vi "电源管理UI.vi"() -> ()   [LabVIEW 2016, in "PLC.lvlib"]
uses:
  PLC.lvlib
  <vilib>/Utility/miscctls.llb/LVPointTypeDef.ctl
panel:
  in  "自动运行启动参数":T1
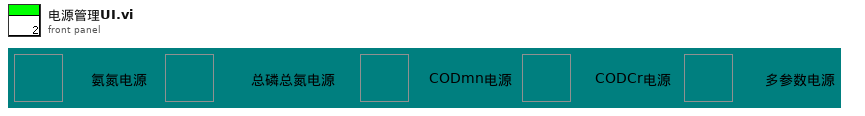
[diagram p1: front panel]
types:
  T1 = cluster{"氨氮":bool, "总磷总氮":bool, "CODmn":bool, "CODCr":bool, "多参数":bool}
  T2 = typedef "LVPointTypeDef.ctl" = cluster{"Horizontal":i16, "Vertical":i16}
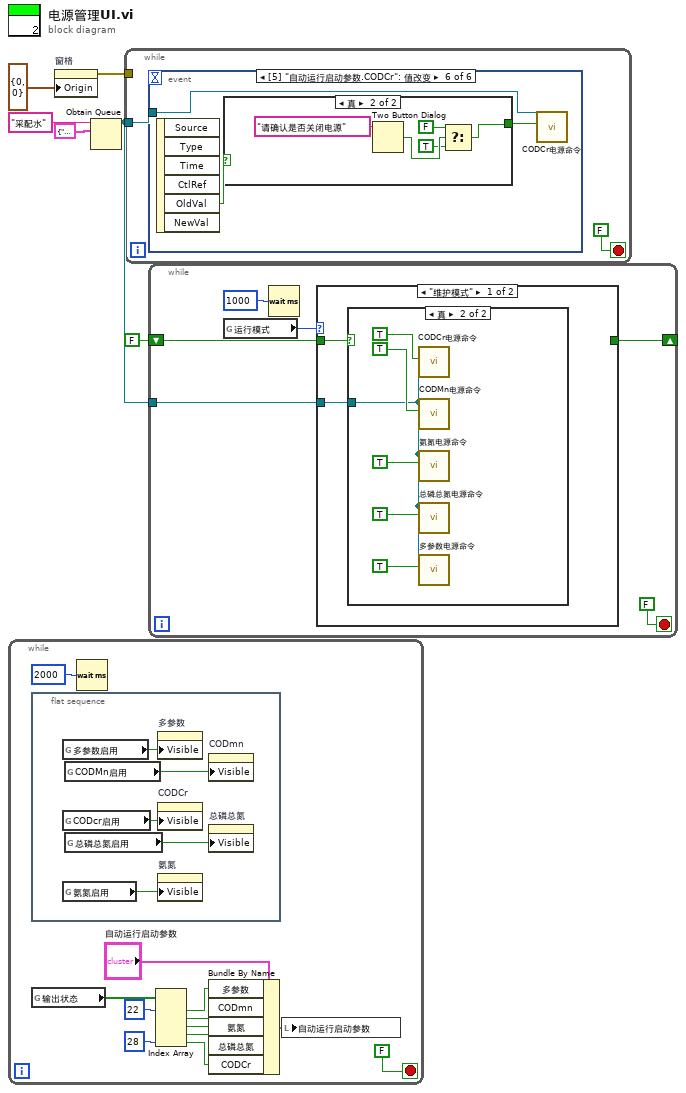
[diagram p0: block diagram]
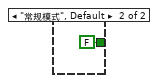
[diagram p3: hidden frame]
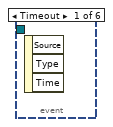
[diagram p4: hidden frame]
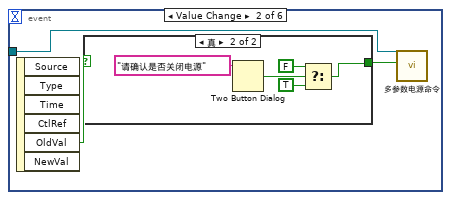
[diagram p5: hidden frame]
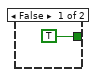
[diagram p6: hidden frame]
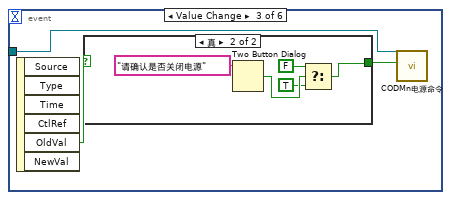
[diagram p7: hidden frame]
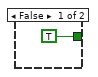
[diagram p8: hidden frame]
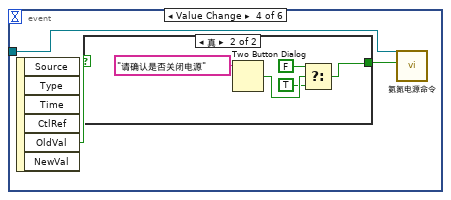
[diagram p9: hidden frame]
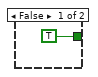
[diagram p10: hidden frame]
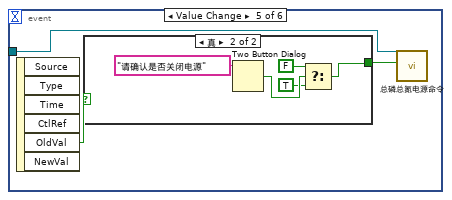
[diagram p11: hidden frame]
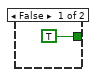
[diagram p12: hidden frame]
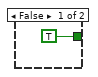
[diagram p13: hidden frame]
diagram:
  n1 = while {
    stop <- FALSE stop-if-true
    n2 = flat-sequence {
      frame #0 {
        n3 = global read "系统设置全局变量.vi" "多参数启用"() -> (w20:bool)
        n4 = global read "系统设置全局变量.vi" "CODcr启用"() -> (w19:bool)
        n5 = global read "系统设置全局变量.vi" "氨氮启用"() -> (w23:bool)
        n6 = global read "系统设置全局变量.vi" "CODMn启用"() -> (w21:bool)
        n7 = global read "系统设置全局变量.vi" "总磷总氮启用"() -> (w22:bool)
        n8 = property on="多参数" class="Bool (严格)"("Visible"=w20) -> ()  [unwired: 2 in, 2 out]
        n9 = property on="CODCr" class="Bool (严格)"("Visible"=w19) -> ()  [unwired: 2 in, 2 out]
        n10 = property on="氨氮" class="Bool (严格)"("Visible"=w23) -> ()  [unwired: 2 in, 2 out]
        n11 = property on="CODmn" class="Bool (严格)"("Visible"=w21) -> ()  [unwired: 2 in, 2 out]
        n12 = property on="总磷总氮" class="Bool (严格)"("Visible"=w22) -> ()  [unwired: 2 in, 2 out]
      }
    }
    n13 = global read "采配水全局变量.vi" "输出状态"() -> (w16:bool[])
    n14 = Wait (ms)(milliseconds to wait=u32 2000 ("等待时间（毫秒）")) -> ()  [unwired: 1 out]
    n15 = Index Array(array=w16, index #1=22 ("索引"), index #5=28 ("索引")) -> (element #1=w12:bool, element #2=w11:bool, element #3=w10:bool, element #4=w9:bool, element #5=w8:bool)  [unwired: 3 in]
    n16 = Bundle By Name(cluster="自动运行启动参数", "多参数"=w12, "CODmn"=w11, "氨氮"=w10, "总磷总氮"=w9, "CODCr"=w8) -> (w7:T1)
    n17 = local write "自动运行启动参数"(w7) -> ()
  }
  n18 = property on="窗格" class="Pane"("Origin"=T2 {"Horizontal"=0, "Vertical"=0} ("原点")) -> (error out=w3:errorcluster)  [unwired: 2 in, 1 out]
  n19 = Obtain Queue(name (unnamed)="采配水" ("名称（未命名）"), element data type=cluster{"命令":string, "数据":variant} {"命令"="", "数据"=variant}) -> (queue out=w2:refnum<queue>)  [unwired: 3 in, 2 out]
  n20 = while {
    tunnel: w2 -> [w24]
    tunnel: w3 -> [_]
    stop <- FALSE stop-if-true
    n21 = event shown="[5] \"自动运行启动参数.CODCr\": 值改变" {
      selector: _ -> [_ _ _ _ _ _]
      dyn-events: _ -> [_ _ _ _ _ _]
      timeout: _ -> [_ _ _ _ _ _]
      tunnel: w24 -> [_ w28 w37 w46 w55 w64]
      event Timeout {
        n22 = event-data() -> ()  [unwired: 1 in, 3 out]
      }
      event "自动运行启动参数.多参数": Value Change {
        n23 = event-data() -> ("OldVal"=w27:bool)  [unwired: 1 in, 5 out]
        n24 = case shown="真" w27 {
          tunnel: [TRUE ("T button?") w30] -> w26
          frame False {
          }
          frame True {
            n25 = Two Button Dialog(message="请确认是否关闭电源" ("消息")) -> (T button?=w33:bool)  [unwired: 2 in]
            n26 = Select(t=FALSE, s=w33, f=TRUE ("T button?")) -> (s? t:f=w30:bool)
          }
        }
        n27 = call "多参数电源命令.vi"("通电/断电"=w26, "队列"=w28) -> ()  [unwired: 9 in, 1 out]
      }
      event "自动运行启动参数.CODmn": Value Change {
        n28 = event-data() -> ("OldVal"=w36:bool)  [unwired: 1 in, 5 out]
        n29 = case shown="真" w36 {
          tunnel: [TRUE ("T button?") w39] -> w35
          frame False {
          }
          frame True {
            n30 = Two Button Dialog(message="请确认是否关闭电源" ("消息")) -> (T button?=w42:bool)  [unwired: 2 in]
            n31 = Select(t=FALSE, s=w42, f=TRUE ("T button?")) -> (s? t:f=w39:bool)
          }
        }
        n32 = call "CODMn电源命令.vi"("通电/断电"=w35, "队列"=w37) -> ()  [unwired: 9 in, 1 out]
      }
      event "自动运行启动参数.氨氮": Value Change {
        n33 = event-data() -> ("OldVal"=w45:bool)  [unwired: 1 in, 5 out]
        n34 = case shown="真" w45 {
          tunnel: [TRUE ("T button?") w48] -> w44
          frame False {
          }
          frame True {
            n35 = Two Button Dialog(message="请确认是否关闭电源" ("消息")) -> (T button?=w51:bool)  [unwired: 2 in]
            n36 = Select(t=FALSE, s=w51, f=TRUE ("T button?")) -> (s? t:f=w48:bool)
          }
        }
        n37 = call "氨氮电源命令.vi"("通电/断电"=w44, "队列"=w46) -> ()  [unwired: 9 in, 1 out]
      }
      event "自动运行启动参数.总磷总氮": Value Change {
        n38 = event-data() -> ("OldVal"=w54:bool)  [unwired: 1 in, 5 out]
        n39 = case shown="真" w54 {
          tunnel: [TRUE ("T button?") w57] -> w53
          frame False {
          }
          frame True {
            n40 = Two Button Dialog(message="请确认是否关闭电源" ("消息")) -> (T button?=w60:bool)  [unwired: 2 in]
            n41 = Select(t=FALSE, s=w60, f=TRUE ("T button?")) -> (s? t:f=w57:bool)
          }
        }
        n42 = call "总磷总氮电源命令.vi"("通电/断电"=w53, "队列"=w55) -> ()  [unwired: 9 in, 1 out]
      }
      event "自动运行启动参数.CODCr": Value Change {
        n43 = event-data() -> ("OldVal"=w63:bool)  [unwired: 1 in, 5 out]
        n44 = case shown="真" w63 {
          tunnel: [TRUE ("T button?") w66] -> w62
          frame False {
          }
          frame True {
            n45 = Two Button Dialog(message="请确认是否关闭电源" ("消息")) -> (T button?=w69:bool)  [unwired: 2 in]
            n46 = Select(t=FALSE, s=w69, f=TRUE ("T button?")) -> (s? t:f=w66:bool)
          }
        }
        n47 = call "CODCr电源命令.vi"("通电/断电"=w62, "队列"=w64) -> ()  [unwired: 9 in, 1 out]
      }
    }
  }
  n48 = while {
    tunnel: w2 -> [w74]
    shift-right: [w71] -> _
    shift-left: FALSE -> [w72]
    stop <- FALSE stop-if-true
    n49 = global read "系统设置全局变量.vi" "运行模式"() -> (w73:enum16{"维护模式", "常规模式", "应急模式", "质控模式"})
    n50 = Wait (ms)(milliseconds to wait=u32 1000 ("等待时间（毫秒）")) -> ()  [unwired: 1 out]
    n51 = case shown="\"维护模式\"" w73 {
      tunnel: w74 -> [w78 _]
      tunnel: w72 -> [w77 _]
      tunnel: [_ FALSE] -> w71
      frame "维护模式" {
        n52 = case shown="真" w77 {
          tunnel: w78 -> [_ w79]
          frame False {
          }
          frame True {
            n53 = call "CODCr电源命令.vi"("通电/断电"=TRUE, "队列"=w79) -> ()  [unwired: 9 in, 1 out]
            n54 = call "CODMn电源命令.vi"("通电/断电"=TRUE, "队列"=w79) -> ()  [unwired: 9 in, 1 out]
            n55 = call "氨氮电源命令.vi"("通电/断电"=TRUE, "队列"=w79) -> ()  [unwired: 9 in, 1 out]
            n56 = call "总磷总氮电源命令.vi"("通电/断电"=TRUE, "队列"=w79) -> ()  [unwired: 9 in, 1 out]
            n57 = call "多参数电源命令.vi"("通电/断电"=TRUE, "队列"=w79) -> ()  [unwired: 9 in, 1 out]
          }
        }
      }
      frame "常规模式", Default {
      }
    }
  }
